vi "Just practice array functions.vi"() -> ()   [LabVIEW 2020]
panel:
  out "array (last n elements first)":dbl[](array[numeric])
  out "second subarray":dbl[](array[numeric])
  out "first subarray":dbl[](array[numeric])
  out "min index(es)":i32
  out "min value":dbl
  out "max index(es)":i32
  out "max value":dbl
  in  "Array 6":dbl[](array[numeric])
  out "subarray":dbl[](array[numeric])
  in  "Array 5":dbl[](array[numeric])
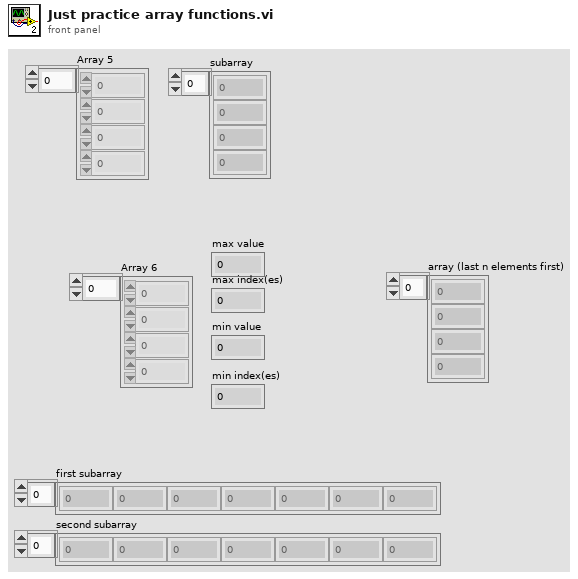
[diagram p1: front panel]
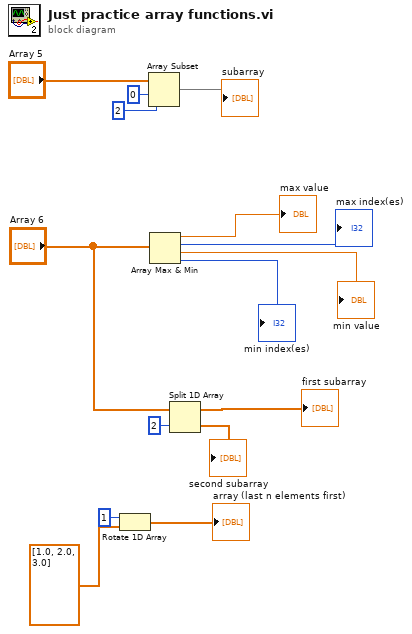
[diagram p0: block diagram]
diagram:
  n1 = Rotate 1D Array(1:dbl[] [1.0, 2.0, 3.0] ("array"), 2:1 ("n")) -> (0:→"array (last n elements first)":dbl[])
  n2 = Array Subset "Array Subset"(array="Array 5", index=0, length=2) -> (→"subarray":dbl[])
  n3 = Array Max & Min(array="Array 6") -> (max value=→"max value":dbl, max index (indices)=→"max index(es)":i32, min value=→"min value":dbl, min index (indices)=→"min index(es)":i32)
  n4 = Split 1D Array(array="Array 6", index=2) -> (first subarray=→"first subarray":dbl[], second subarray=→"second subarray":dbl[])
